vi "CRYView Outing_CurLibrary.vi"() -> ()   [LabVIEW 2013]
uses:
  SubVI/CRYMain Sub Window Global.vi
  CRYView Global.vi
panel:
  in  "bUpdateAllView":bool
  in  "bDropReport":bool
  in  "bGetGraphData":bool
  in  "bSetGraphData":bool
  in  "bSend":bool
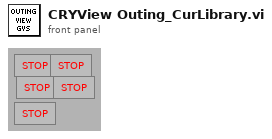
[diagram p1: front panel]
types:
  T1 = cluster{"sAction":string, "sData":string, "nData":i32, "pVIRef":refnum<vi>}
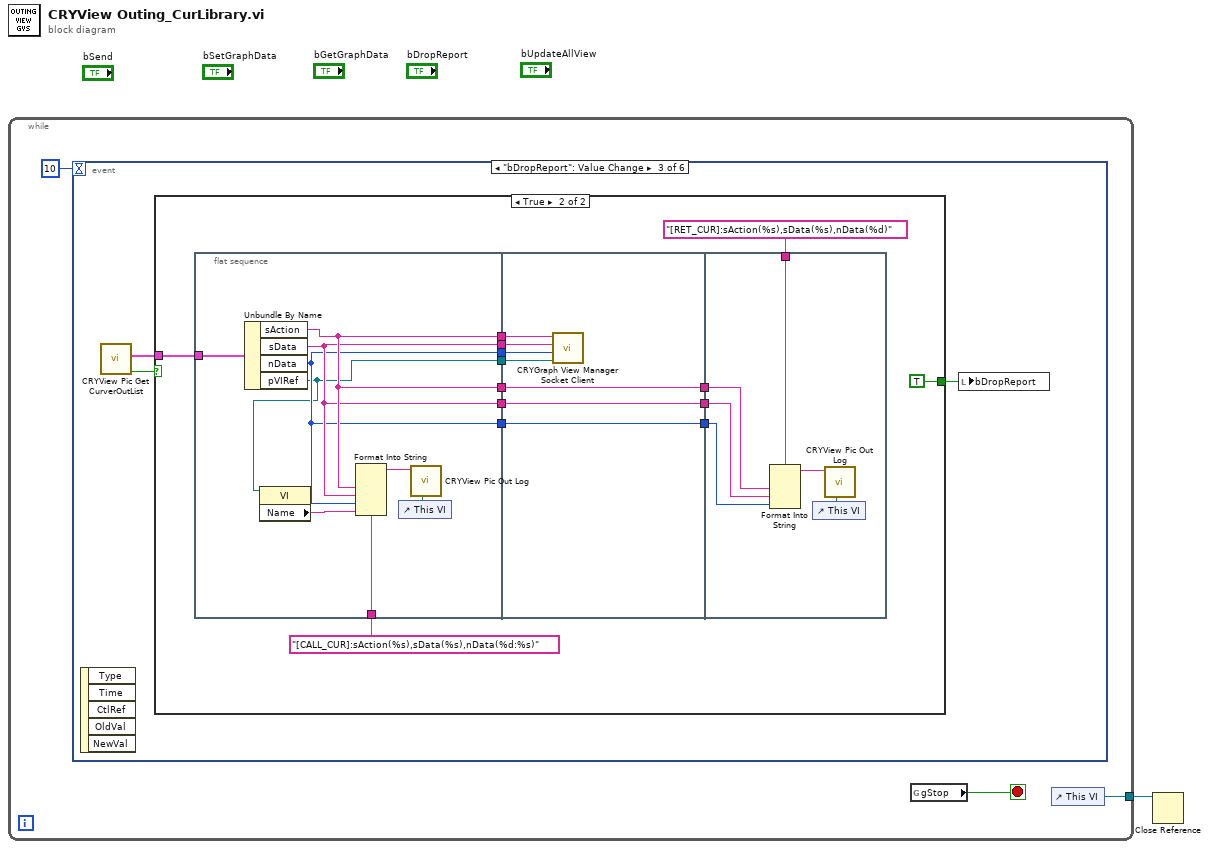
[diagram p0: block diagram]
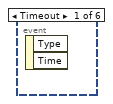
[diagram p2: hidden frame]
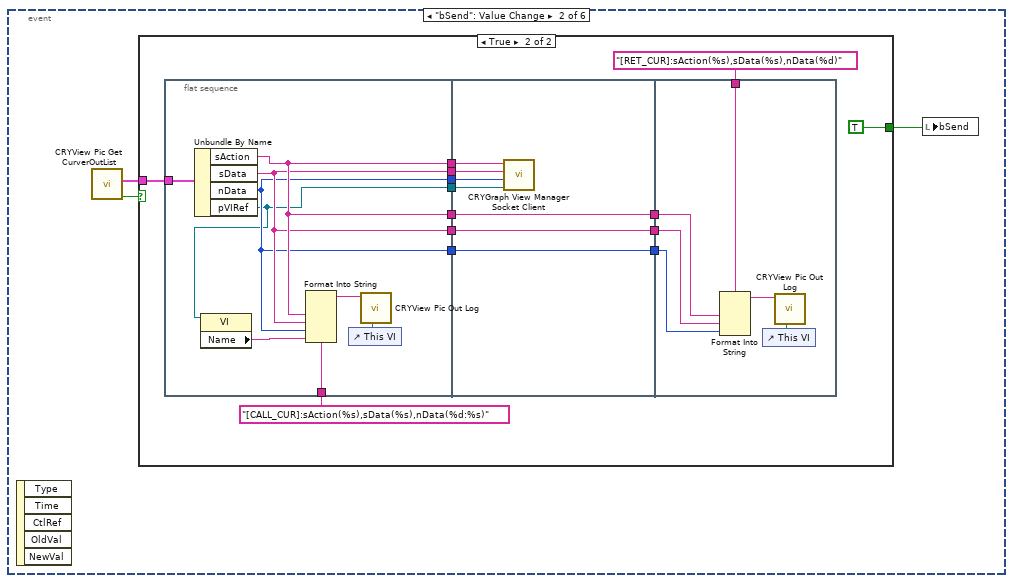
[diagram p3: hidden frame]
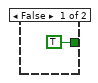
[diagram p4: hidden frame]
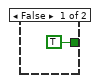
[diagram p5: hidden frame]
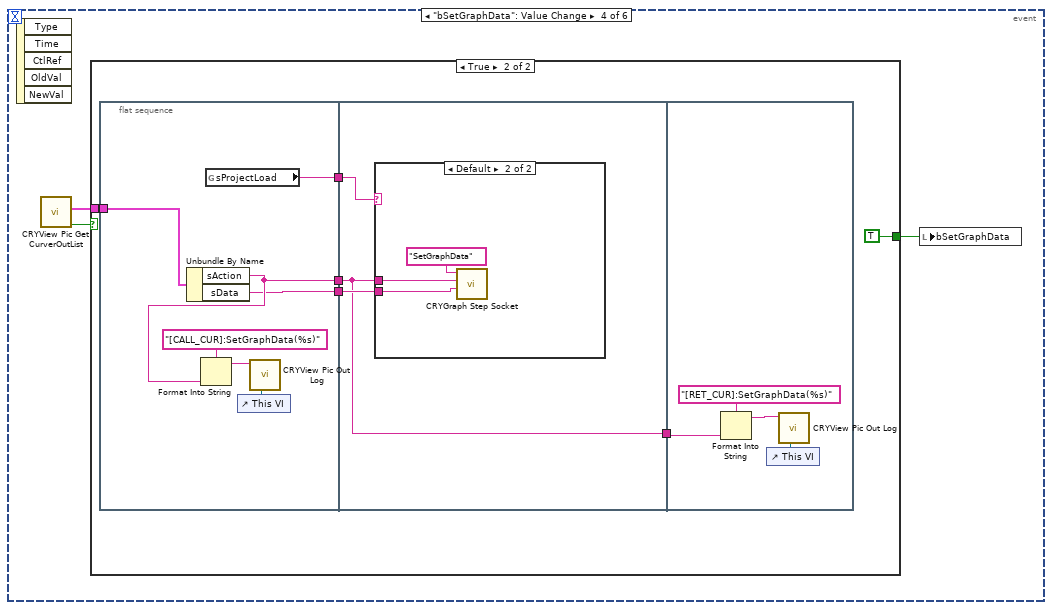
[diagram p6: hidden frame]
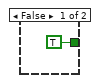
[diagram p7: hidden frame]
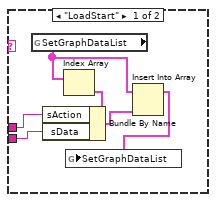
[diagram p8: hidden frame]
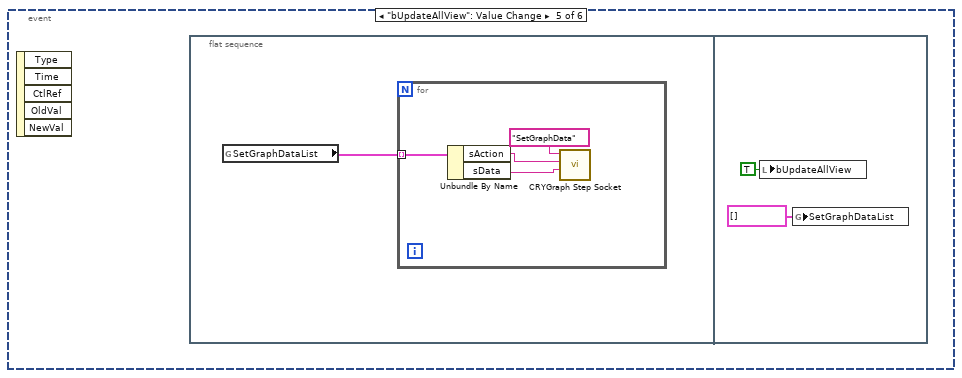
[diagram p9: hidden frame]
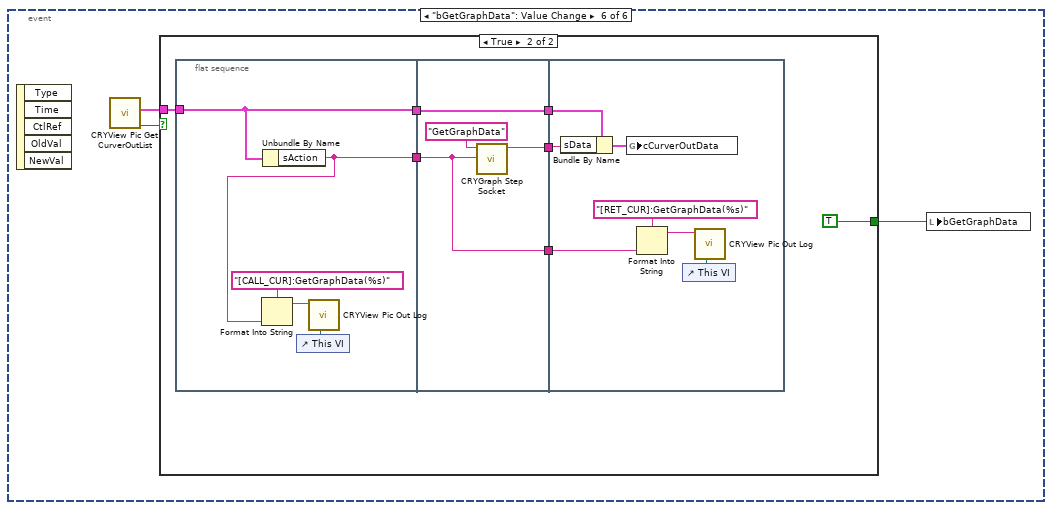
[diagram p10: hidden frame]
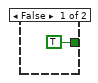
[diagram p11: hidden frame]
diagram:
  n1 = while {
    tunnel: [w4] -> w1
    stop <- w3 stop-if-true
    n2 = event shown="[2] \"bDropReport\": Value Change" {
      selector: _ -> [_ _ _ _ _ _]
      dyn-events: _ -> [_ _ _ _ _ _]
      timeout: 10 -> [_ _ _ _ _ _]
      event Timeout {
        n3 = event-data() -> ()  [unwired: 1 in, 2 out]
      }
      event "bSend": Value Change {
        n4 = event-data() -> ()  [unwired: 1 in, 5 out]
        n5 = call "CRYView Pic Get CurverOutList.vi"() -> ("bResult"=w5:bool, "cCurverOutData_Out"=w6:T1)  [unwired: 10 in]
        n6 = case shown="True" w5 {
          tunnel: [TRUE ("StateOut") TRUE ("StateOut")] -> w7
          tunnel: w6 -> [_ w9]
          frame False {
          }
          frame True {
            n7 = flat-sequence {
              tunnel: [w28] -> w22
              tunnel: [w27] -> w21
              tunnel: [w26] -> w20
              tunnel: [w28] -> w19
              tunnel: [w27] -> w18
              tunnel: [w26] -> w17
              tunnel: [w25] -> w16
              tunnel: "[CALL_CUR]:sAction(%s),sData(%s),nData(%d:%s)" ("format string") -> [w24]
              tunnel: w9 -> [w23]
              tunnel: w22 -> [w38]
              tunnel: [w38] -> w15
              tunnel: w21 -> [w37]
              tunnel: [w37] -> w14
              tunnel: w20 -> [w36]
              tunnel: [w36] -> w13
              tunnel: w19 -> [w35]
              tunnel: w18 -> [w34]
              tunnel: w17 -> [w33]
              tunnel: w16 -> [w32]
              tunnel: w15 -> [w42]
              tunnel: w14 -> [w41]
              tunnel: w13 -> [w40]
              tunnel: "[RET_CUR]:sAction(%s),sData(%s),nData(%d)" ("format string") -> [w39]
              frame #0 {
                n8 = Unbundle By Name(w23) -> ("sAction"=w28:string, "sData"=w27:string, "nData"=w26:i32, "pVIRef"=w25:refnum<vi>)
                n9 = property class="VI"(reference=w25) -> ("Name"=w29:string)  [unwired: 1 in, 2 out]
                n10 = Format Into String(format string=w24, w28, w27, w26, w29) -> (resulting string=w31:string)  [unwired: 2 in, 1 out]
                n11 = control-ref of="This VI"() -> (w30:refnum<vi>)
                n12 = call "CRYView Pic Out Log.vi"("vi reference"=w30, "sData"=w31) -> ()  [unwired: 10 in]
              }
              frame #1 {
                n13 = call "CRYGraph View Manager Socket Client.vi"("pVI Ref"=w32, "nData"=w33, "sData"=w34, "sAction"=w35) -> ()  [unwired: 8 in]
              }
              frame #2 {
                n14 = Format Into String(format string=w39, w42, w41, w40) -> (resulting string=w43:string)  [unwired: 2 in, 1 out]
                n15 = control-ref of="This VI"() -> (w44:refnum<vi>)
                n16 = call "CRYView Pic Out Log.vi"("vi reference"=w44, "sData"=w43) -> ()  [unwired: 10 in]
              }
            }
          }
        }
        n17 = local write "bSend"(w7) -> ()
      }
      event "bDropReport": Value Change {
        n18 = event-data() -> ()  [unwired: 1 in, 5 out]
        n19 = call "CRYView Pic Get CurverOutList.vi"() -> ("bResult"=w46:bool, "cCurverOutData_Out"=w47:T1)  [unwired: 10 in]
        n20 = case shown="True" w46 {
          tunnel: w47 -> [_ w50]
          tunnel: [TRUE ("StateOut") TRUE ("StateOut")] -> w45
          frame False {
          }
          frame True {
            n21 = flat-sequence {
              tunnel: [w68] -> w62
              tunnel: [w67] -> w61
              tunnel: [w66] -> w60
              tunnel: [w68] -> w59
              tunnel: [w67] -> w58
              tunnel: [w66] -> w57
              tunnel: [w65] -> w56
              tunnel: "[CALL_CUR]:sAction(%s),sData(%s),nData(%d:%s)" ("format string") -> [w64]
              tunnel: w50 -> [w63]
              tunnel: w62 -> [w78]
              tunnel: [w78] -> w55
              tunnel: w61 -> [w77]
              tunnel: [w77] -> w54
              tunnel: w60 -> [w76]
              tunnel: [w76] -> w53
              tunnel: w59 -> [w75]
              tunnel: w58 -> [w74]
              tunnel: w57 -> [w73]
              tunnel: w56 -> [w72]
              tunnel: w55 -> [w82]
              tunnel: w54 -> [w81]
              tunnel: w53 -> [w80]
              tunnel: "[RET_CUR]:sAction(%s),sData(%s),nData(%d)" ("format string") -> [w79]
              frame #0 {
                n22 = Unbundle By Name(w63) -> ("sAction"=w68:string, "sData"=w67:string, "nData"=w66:i32, "pVIRef"=w65:refnum<vi>)
                n23 = property class="VI"(reference=w65) -> ("Name"=w69:string)  [unwired: 1 in, 2 out]
                n24 = Format Into String(format string=w64, w68, w67, w66, w69) -> (resulting string=w71:string)  [unwired: 2 in, 1 out]
                n25 = control-ref of="This VI"() -> (w70:refnum<vi>)
                n26 = call "CRYView Pic Out Log.vi"("vi reference"=w70, "sData"=w71) -> ()  [unwired: 10 in]
              }
              frame #1 {
                n27 = call "CRYGraph View Manager Socket Client.vi"("pVI Ref"=w72, "nData"=w73, "sData"=w74, "sAction"=w75) -> ()  [unwired: 8 in]
              }
              frame #2 {
                n28 = Format Into String(format string=w79, w82, w81, w80) -> (resulting string=w83:string)  [unwired: 2 in, 1 out]
                n29 = control-ref of="This VI"() -> (w84:refnum<vi>)
                n30 = call "CRYView Pic Out Log.vi"("vi reference"=w84, "sData"=w83) -> ()  [unwired: 10 in]
              }
            }
          }
        }
        n31 = local write "bDropReport"(w45) -> ()
      }
      event "bSetGraphData": Value Change {
        n32 = event-data() -> ()  [unwired: 1 in, 5 out]
        n33 = call "CRYView Pic Get CurverOutList.vi"() -> ("bResult"=w85:bool, "cCurverOutData_Out"=w86:T1)  [unwired: 10 in]
        n34 = case shown="True" w85 {
          tunnel: [TRUE ("bSetGraphData_Out") TRUE ("bSetGraphData_Out")] -> w87
          tunnel: w86 -> [_ w89]
          frame False {
          }
          frame True {
            n35 = flat-sequence {
              tunnel: [w98] -> w94
              tunnel: [w97] -> w93
              tunnel: [w96] -> w92
              tunnel: w89 -> [w95]
              tunnel: [w103] -> w91
              tunnel: w94 -> [w103]
              tunnel: w93 -> [w104]
              tunnel: w92 -> [w102]
              tunnel: w91 -> [w114]
              frame #0 {
                n36 = Unbundle By Name(w95) -> ("sAction"=w98:string, "sData"=w97:string)
                n37 = Format Into String(format string="[CALL_CUR]:SetGraphData(%s)", w98) -> (resulting string=w101:string)  [unwired: 2 in, 1 out]
                n38 = global read "CRYMain Sub Window Global.vi" "sProjectLoad"() -> (w96:string)
                n39 = control-ref of="This VI"() -> (w99:refnum<vi>)
                n40 = call "CRYView Pic Out Log.vi"("vi reference"=w99, "sData"=w101) -> ()  [unwired: 10 in]
              }
              frame #1 {
                n41 = case shown="Default" w102 {
                  tunnel: w104 -> [w108 w113]
                  tunnel: w103 -> [w109 w112]
                  frame "LoadStart" {
                    n42 = global read "CRYView Global.vi" "SetGraphDataList"() -> (w107:cluster{"sAction":string, "sData":string}[])
                    n43 = Index Array(array=w107) -> (element=w110:cluster{"sAction":string, "sData":string})  [unwired: 1 in]
                    n44 = Bundle By Name(cluster=w110, "sAction"=w109, "sData"=w108) -> (w106:cluster{"sAction":string, "sData":string})
                    n45 = Insert Into Array(array=w107, new element=w106) -> (w105:cluster{"sAction":string, "sData":string}[])  [unwired: 1 in]
                    n46 = global write "CRYView Global.vi" "SetGraphDataList"(w105) -> ()
                  }
                  frame Default {
                    n47 = call "CRYGraph Step Socket.vi"("sData"=w113, "Queue Name"=w112, "sAction"="SetGraphData") -> ()  [unwired: 8 in, 1 out]
                  }
                }
              }
              frame #2 {
                n48 = Format Into String(format string="[RET_CUR]:SetGraphData(%s)", w114) -> (resulting string=w115:string)  [unwired: 2 in, 1 out]
                n49 = control-ref of="This VI"() -> (w117:refnum<vi>)
                n50 = call "CRYView Pic Out Log.vi"("vi reference"=w117, "sData"=w115) -> ()  [unwired: 10 in]
              }
            }
          }
        }
        n51 = local write "bSetGraphData"(w87) -> ()
      }
      event "bUpdateAllView": Value Change {
        n52 = event-data() -> ()  [unwired: 1 in, 5 out]
        n53 = flat-sequence {
          frame #0 {
            n54 = global read "CRYView Global.vi" "SetGraphDataList"() -> (w118:cluster{"sAction":string, "sData":string}[])
            n55 = for {
              tunnel: w118 -> [w121] mode=indexing
              n56 = Unbundle By Name(w121) -> ("sAction"=w120:string, "sData"=w119:string)
              n57 = call "CRYGraph Step Socket.vi"("sData"=w119, "Queue Name"=w120, "sAction"="SetGraphData") -> ()  [unwired: 8 in, 1 out]
            }
          }
          frame #1 {
            n58 = local write "bUpdateAllView"(TRUE ("bUpdateAllView")) -> ()
            n59 = global write "CRYView Global.vi" "SetGraphDataList"(cluster{"sAction":string, "sData":string}[] [] ("SetGraphDataList")) -> ()
          }
        }
      }
      event "bGetGraphData": Value Change {
        n60 = event-data() -> ()  [unwired: 1 in, 5 out]
        n61 = call "CRYView Pic Get CurverOutList.vi"() -> ("bResult"=w125:bool, "cCurverOutData_Out"=w126:T1)  [unwired: 10 in]
        n62 = case shown="True" w125 {
          tunnel: [TRUE ("bSetGraphData_Out") TRUE ("bSetGraphData_Out")] -> w127
          tunnel: w126 -> [_ w129]
          frame False {
          }
          frame True {
            n63 = flat-sequence {
              tunnel: [w136] -> w135
              tunnel: [w137] -> w134
              tunnel: w129 -> [w136]
              tunnel: [w141] -> w133
              tunnel: [w142] -> w132
              tunnel: w135 -> [w144]
              tunnel: [w144] -> w131
              tunnel: w134 -> [w141]
              tunnel: w133 -> [w148]
              tunnel: w132 -> [w146]
              tunnel: w131 -> [w147]
              frame #0 {
                n64 = Unbundle By Name(w136) -> ("sAction"=w137:string)
                n65 = Format Into String(format string="[CALL_CUR]:GetGraphData(%s)", w137) -> (resulting string=w140:string)  [unwired: 2 in, 1 out]
                n66 = control-ref of="This VI"() -> (w138:refnum<vi>)
                n67 = call "CRYView Pic Out Log.vi"("vi reference"=w138, "sData"=w140) -> ()  [unwired: 10 in]
              }
              frame #1 {
                n68 = call "CRYGraph Step Socket.vi"("Queue Name"=w141, "sAction"="GetGraphData") -> ("sDataOut"=w142:string)  [unwired: 9 in]
              }
              frame #2 {
                n69 = Bundle By Name(cluster=w147, "sData"=w146) -> (w145:T1)
                n70 = global write "CRYView Global.vi" "cCurverOutData"(w145) -> ()
                n71 = Format Into String(format string="[RET_CUR]:GetGraphData(%s)", w148) -> (resulting string=w149:string)  [unwired: 2 in, 1 out]
                n72 = control-ref of="This VI"() -> (w151:refnum<vi>)
                n73 = call "CRYView Pic Out Log.vi"("vi reference"=w151, "sData"=w149) -> ()  [unwired: 10 in]
              }
            }
          }
        }
        n74 = local write "bGetGraphData"(w127) -> ()
      }
    }
    n75 = global read "CRYMain Sub Window Global.vi" "gStop"() -> (w3:bool)
    n76 = control-ref of="This VI"() -> (w4:refnum<vi>)
  }
  n77 = Close Reference(reference=w1) -> ()  [unwired: 1 in, 1 out]
